vi "Model.vi"(0 "reference in":refnum<class "Battery.lvclass">, 5 "error in":errorcluster) -> (14 "reference out":refnum<class "Battery.lvclass">, 19 "error out":errorcluster)   [LabVIEW 2023, in "Battery.lvclass"]
uses:
  Battery.lvclass
  <vilib>/Utility/SystemLogging/NI_SystemLogging.lvlib
panel:
  out "Chart":dbl[][](graph)
  out "MODE":T1(ring)
  out "MODEL INDEX":i32
  out "error info":errorcluster
  out "Last Command":string
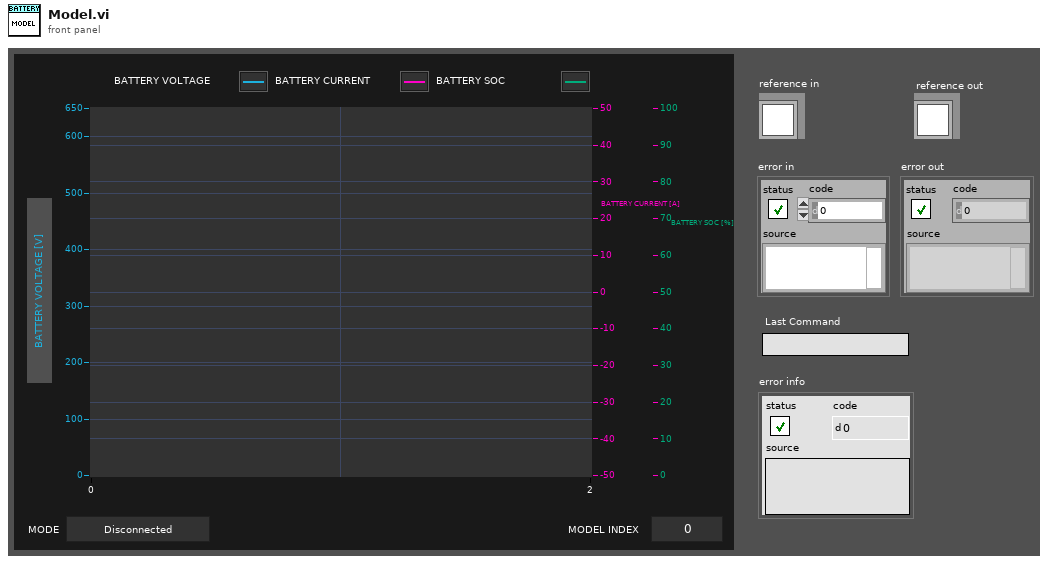
[diagram p1: front panel]
types:
  T1 = enum16{"Disconnected", "Charging", "Discharging"}
  T2 = cluster{"Core":cluster{"Timeout":i32, "Events":cluster{"EventsToProcess":refnum<event-registration>}, "EventFromProcess":refnum<user-event>, "ProcessSyncQueue":refnum<queue>, "QueueFromProcess":refnum<queue>, "Command":string, "Data":variant}}
  T3 = enum32{"Invalid", "Standard", "Closed", "Hidden", "Minimized", "Maximized"}
  T4 = cluster{"EventsToProcess":refnum<event-registration>}
  T5 = typedef "Battery.lvclass/ObjectAttributes.ctl" = cluster{"Mode":enum16{"Disconnected", "Charging", "Discharging"}, "Discharge Switch":bool, "Cell Voltage (V)":dbl, "Cell Current (A)":dbl, "SoC (%)":dbl, "Nominal Voltage (V)":dbl, "Model Index":i32}
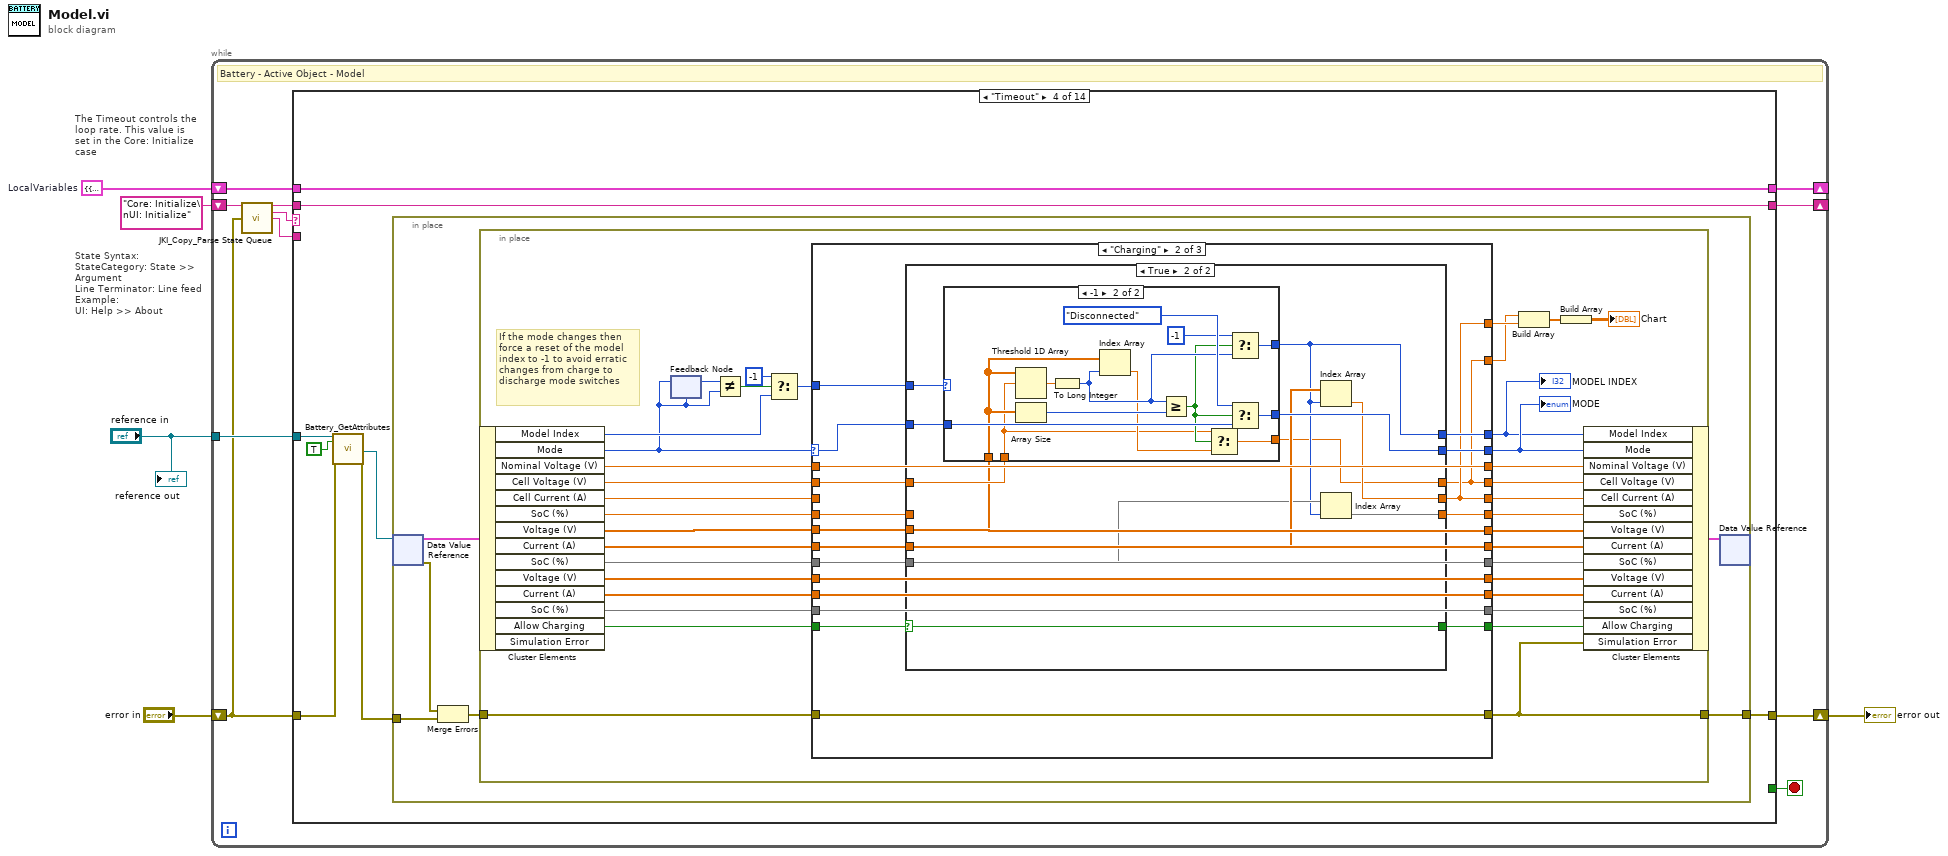
[diagram p0: block diagram]
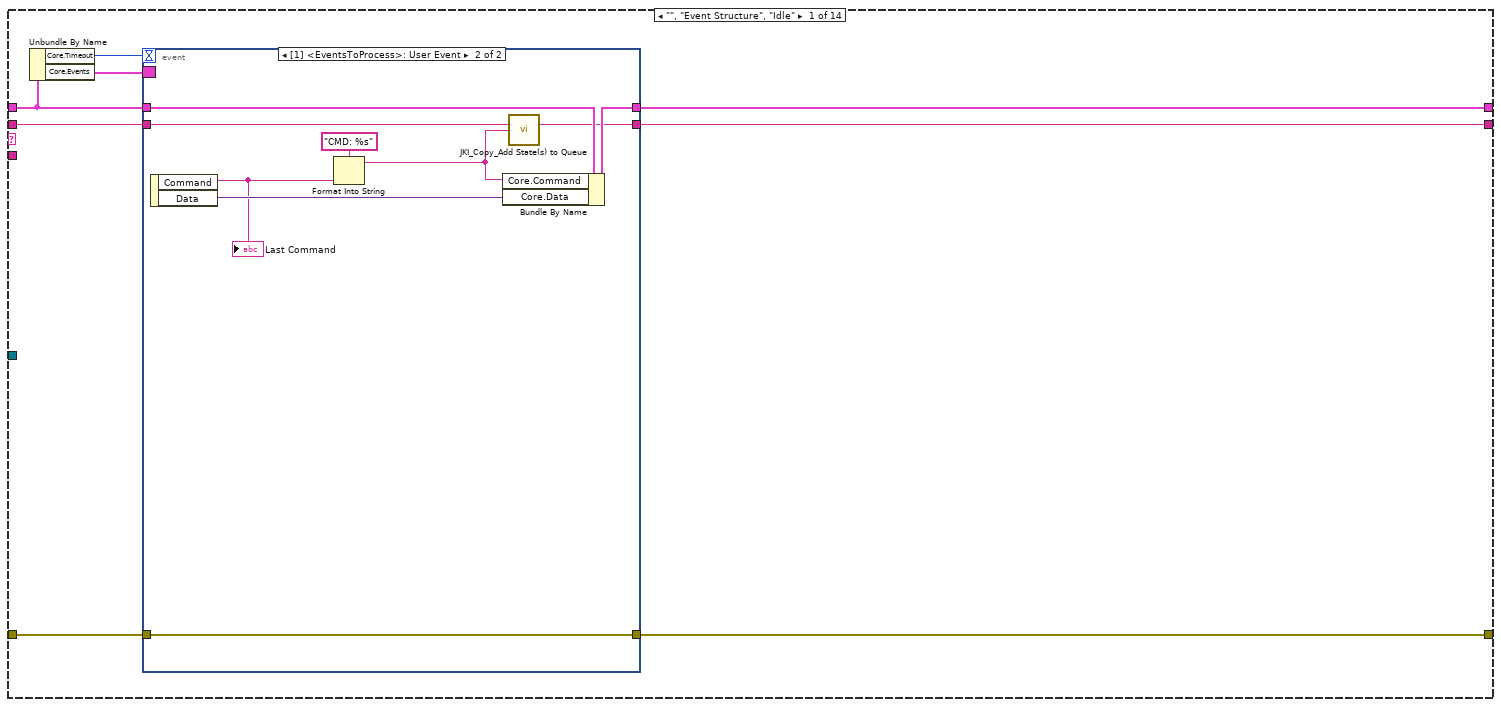
[diagram p2: hidden frame]
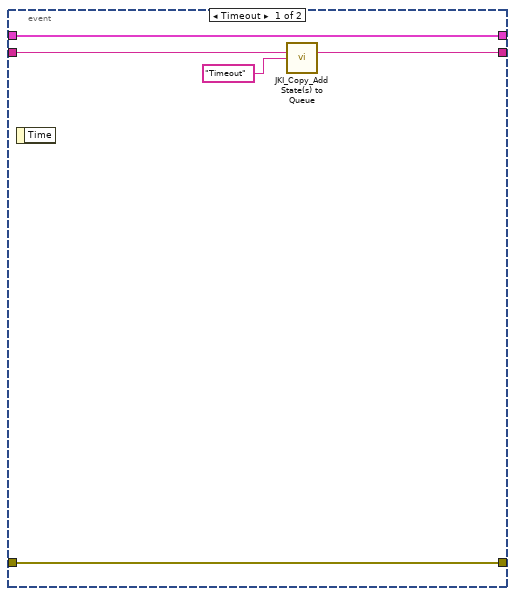
[diagram p3: hidden frame]
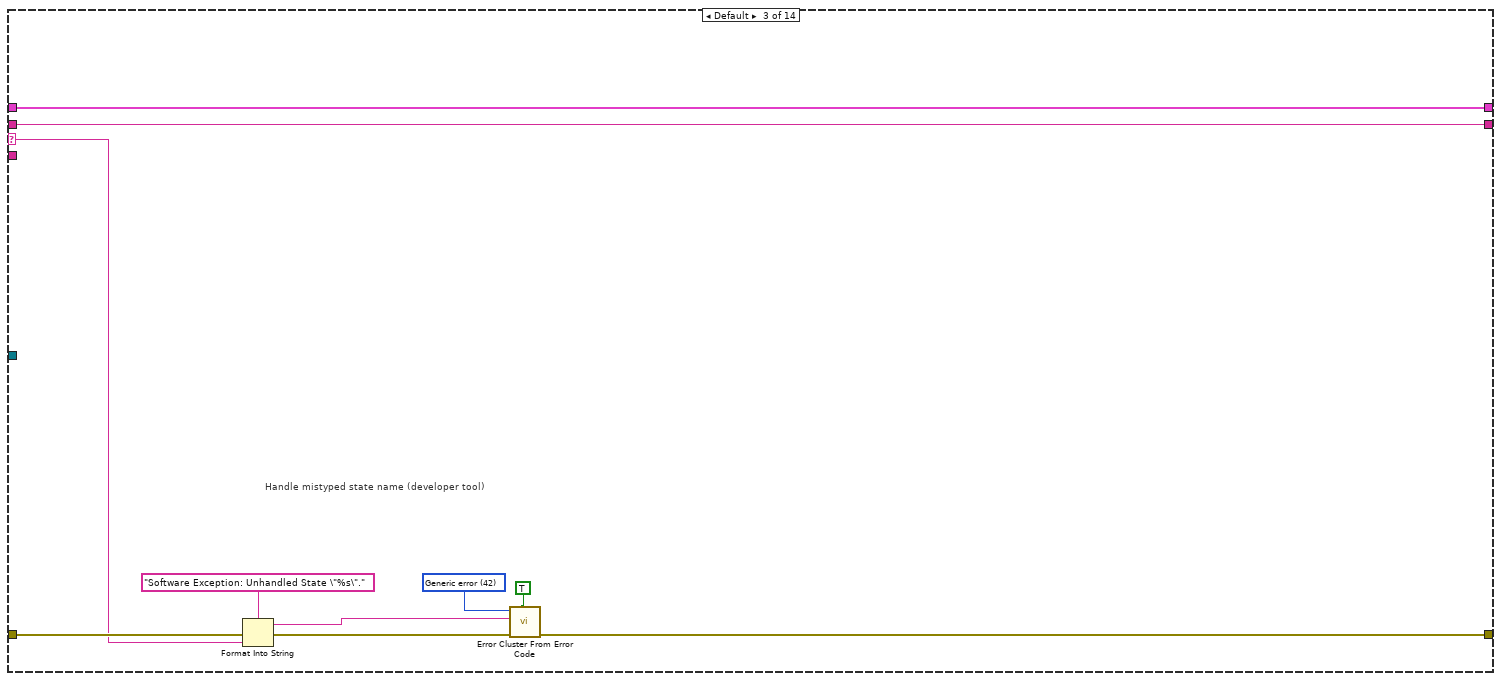
[diagram p5: hidden frame]
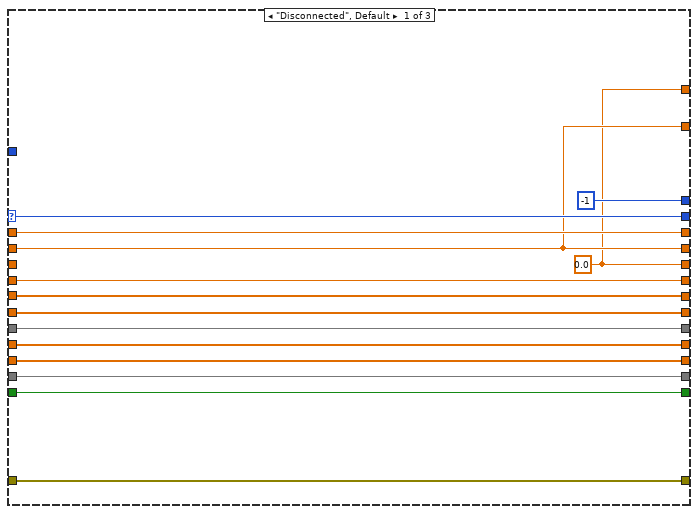
[diagram p6: hidden frame]
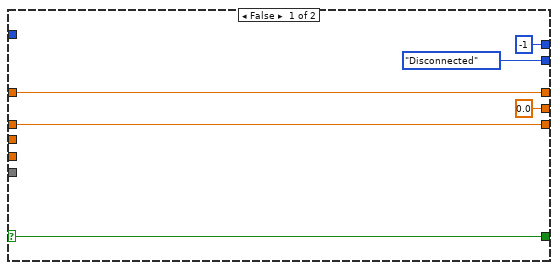
[diagram p7: hidden frame]
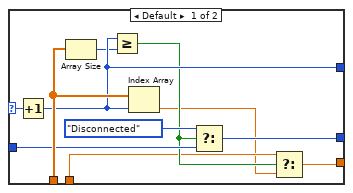
[diagram p8: hidden frame]
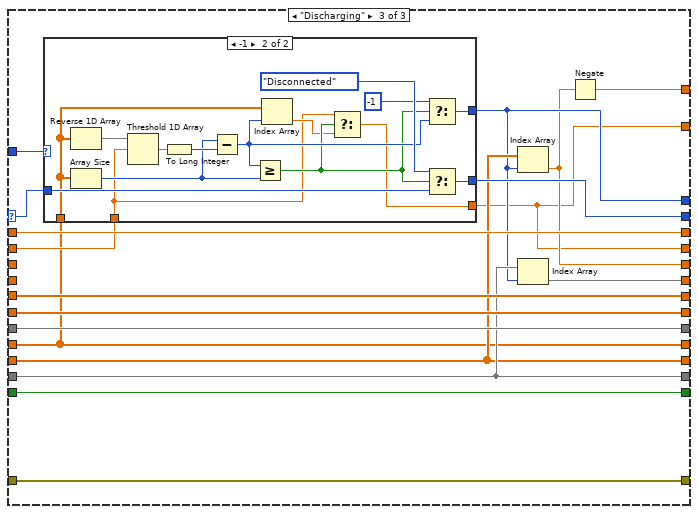
[diagram p9: hidden frame]
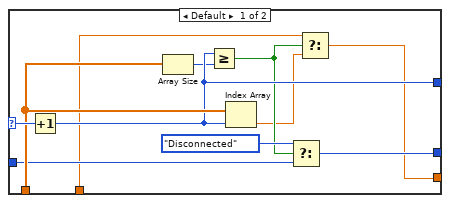
[diagram p10: hidden frame]
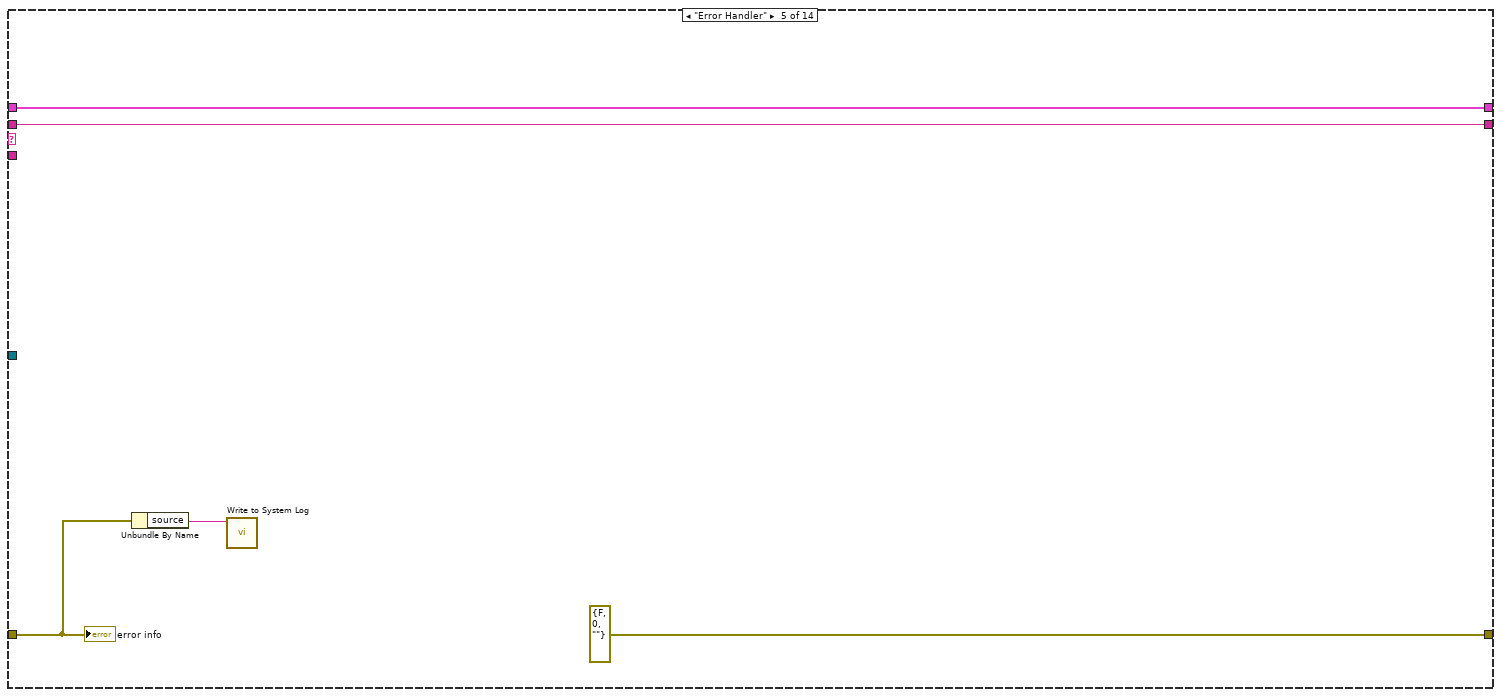
[diagram p11: hidden frame]
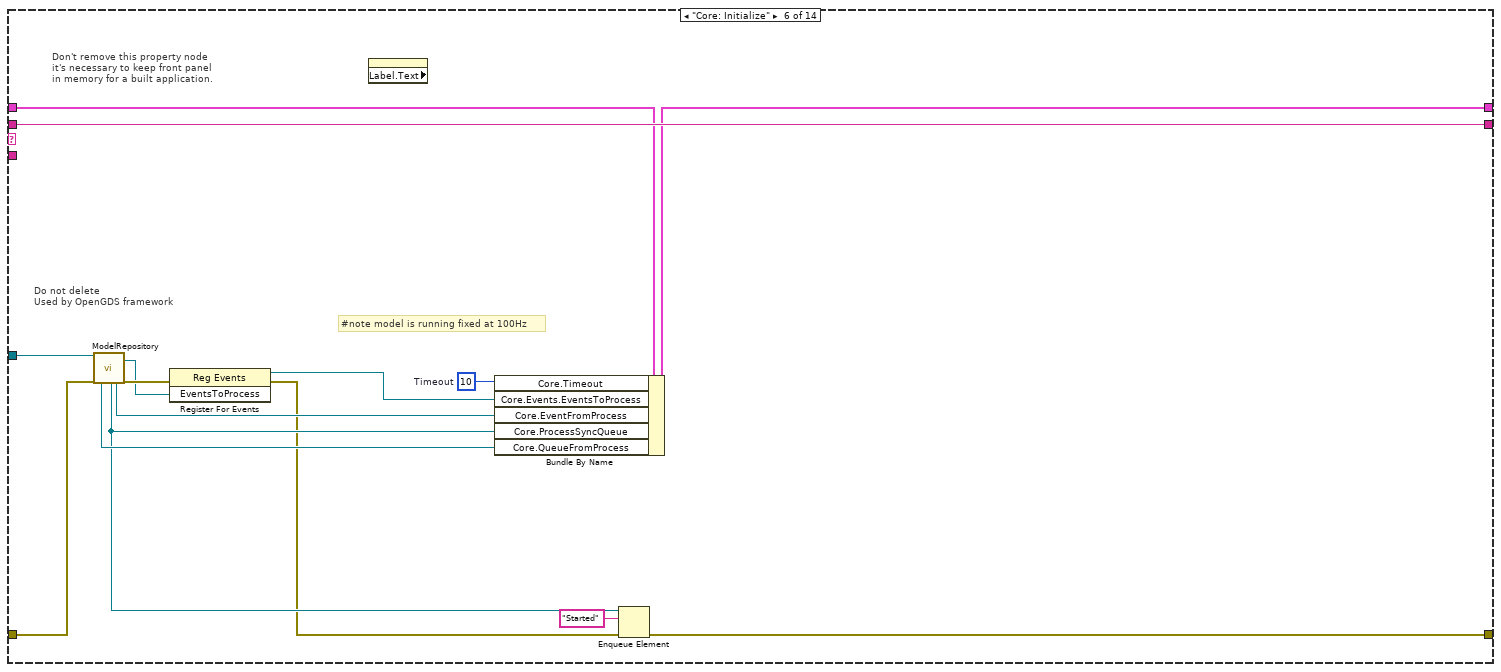
[diagram p12: hidden frame]
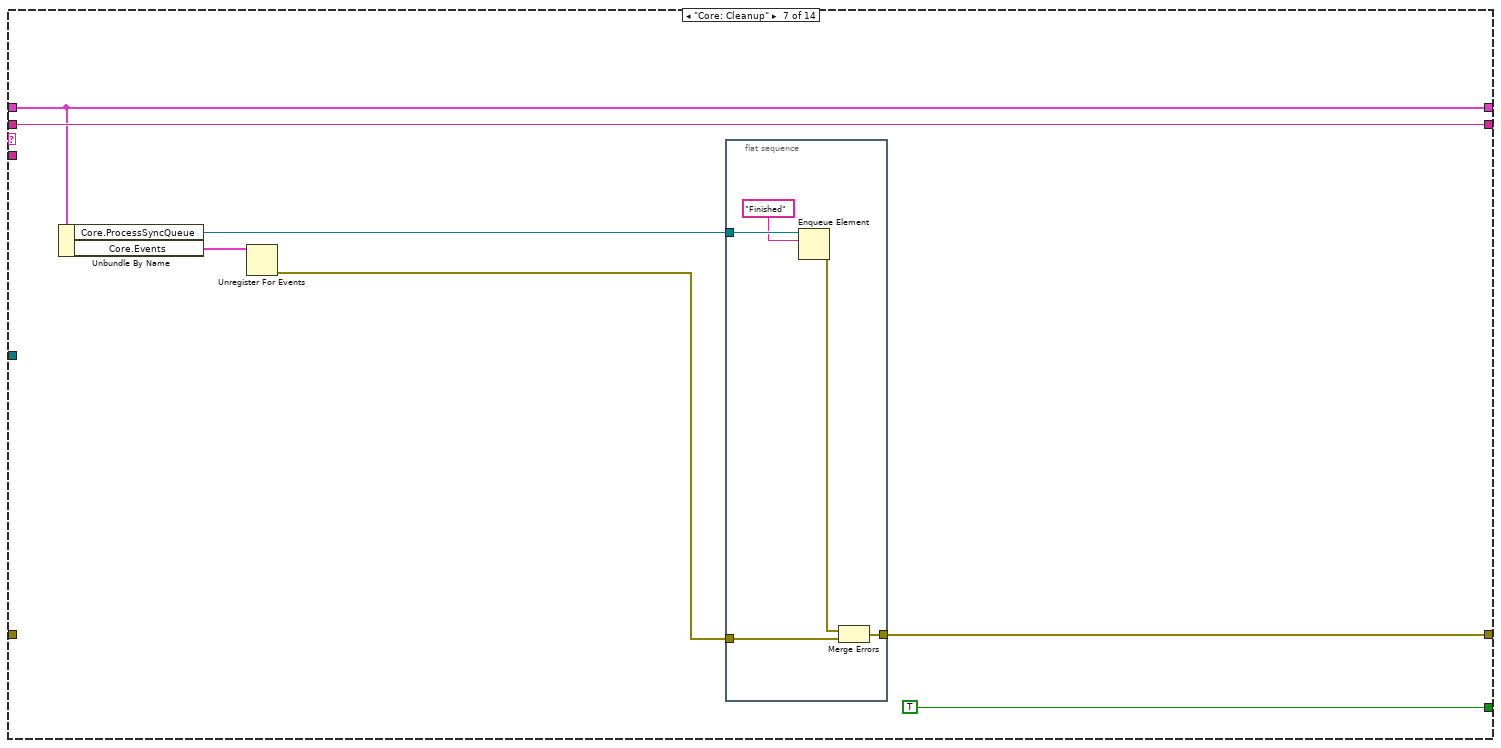
[diagram p13: hidden frame]
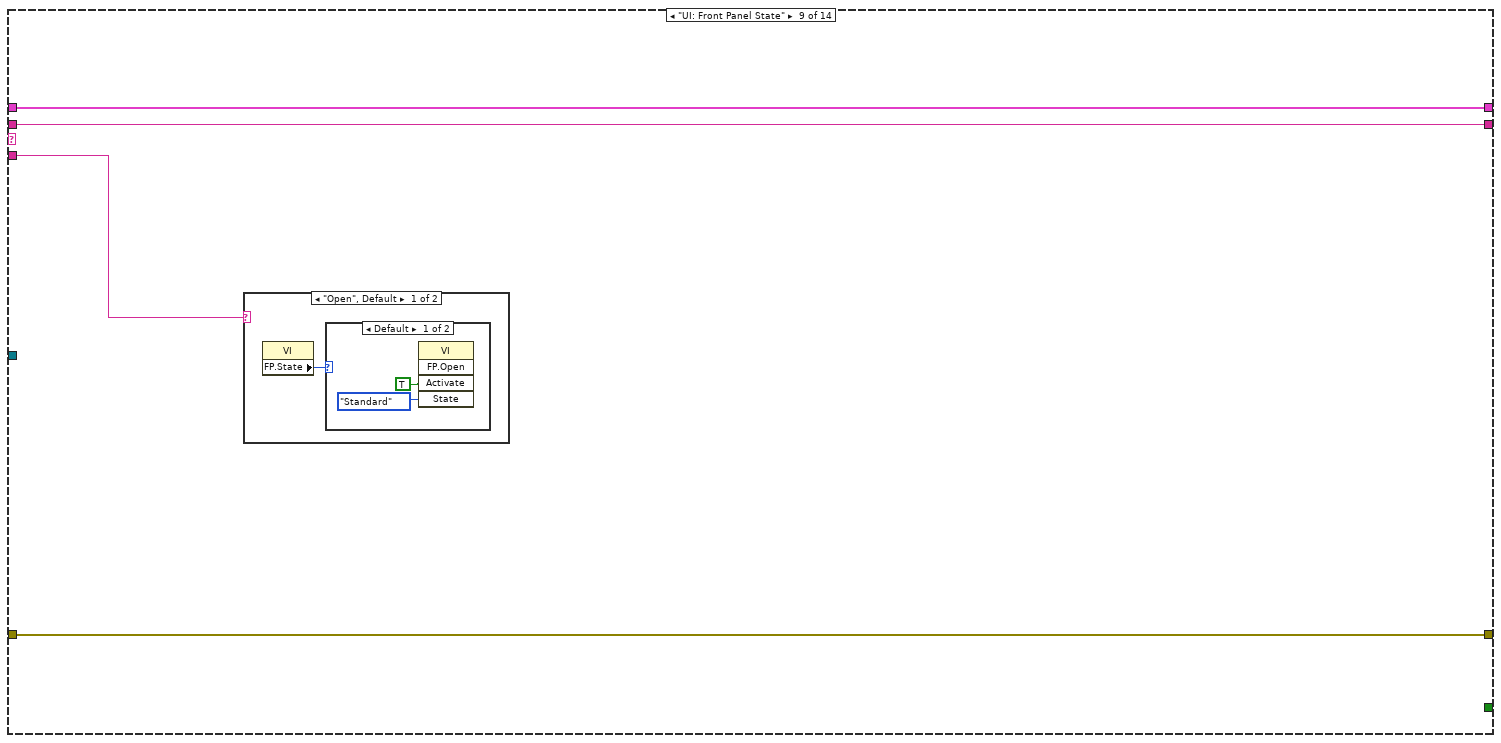
[diagram p15: hidden frame]
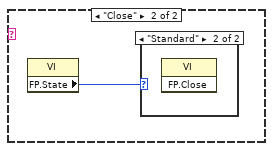
[diagram p17: hidden frame]
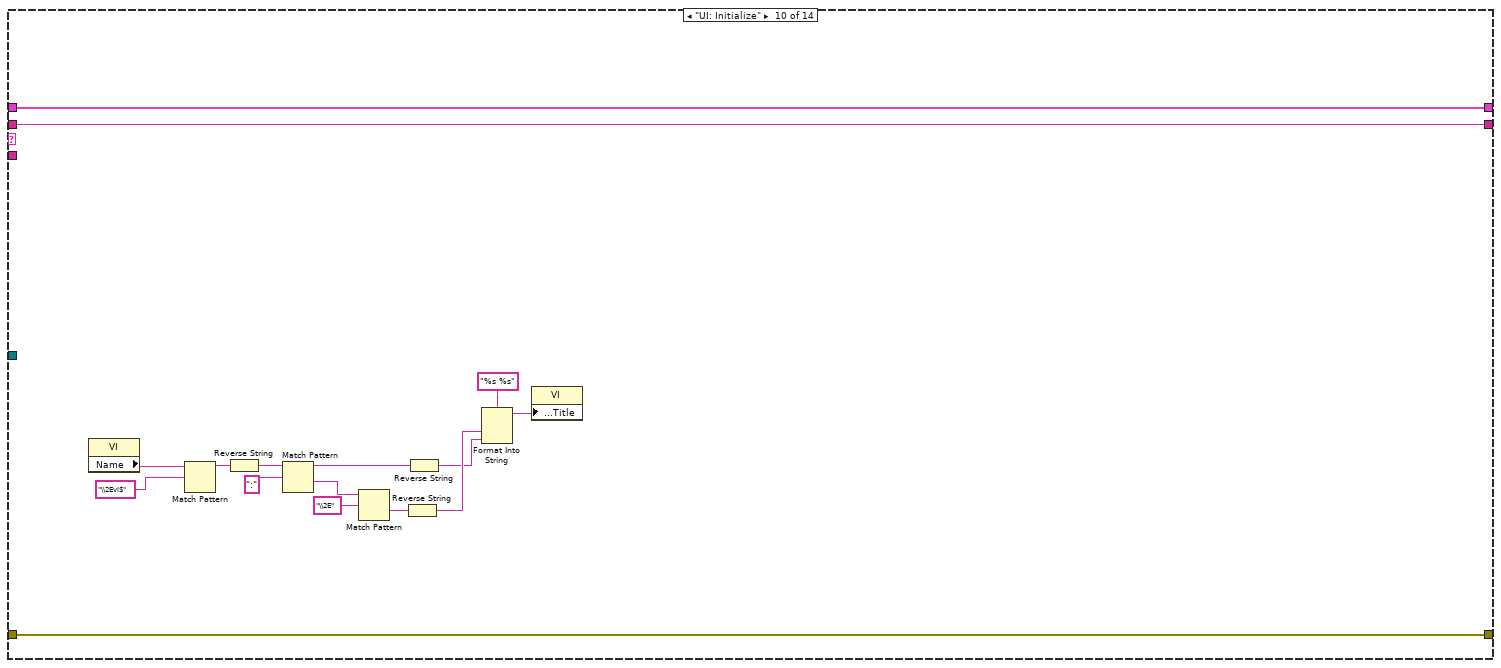
[diagram p19: hidden frame]
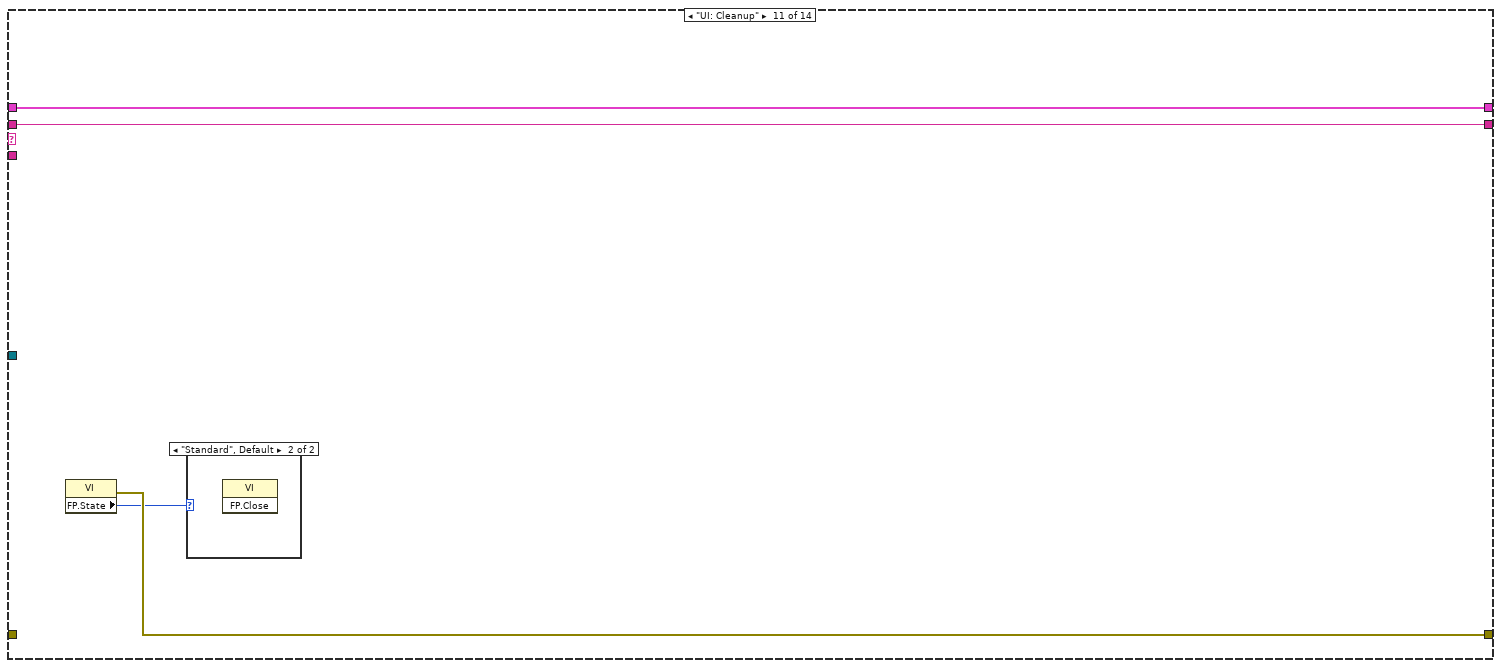
[diagram p20: hidden frame]
diagram:
  w5 = T2 {"Core"={"Timeout"=-1, "Events"={"EventsToProcess"=refnum}, "EventFromProcess"=refnum, "ProcessSyncQueue"=refnum, "QueueFromProcess"=refnum, "Command"="", "Data"=variant}}  # LocalVariables
  # "State Syntax:\nStateCategory: State >> Argument\nLine Terminator: Line feed\nExample:\nUI: Help >> About"
  # "The Timeout controls the loop rate. This value is set in the Core: Initialize case"
  n1 = while {
    shift-right: [w16] -> w4
    shift-left: "error in" -> [w6]
    shift-right: [w13] -> _
    shift-left: "Core: Initialize\nUI: Initialize" ("States Out") -> [w10]
    shift-right: [w15] -> _
    shift-left: w5 -> [w14]
    tunnel: "reference in" -> [w11]
    stop <- w12 stop-if-true
    # "Battery - Active Object - Model"
    n2 = call <vilib>:"JKI_Copy_Parse State Queue.vi"("State Queue"=w10, "Error In (no error)"=w6) -> ("Remaining States"=w9:string, "Current State"=w7:string, "Arguments"=w8:string)  [unwired: 11 in]
    n3 = case shown="\"Timeout\"" w7 {
      selector: w7 -> [_ _ w42 _ _ _ _ _ _ _ _ _ _ _]
      tunnel: w6 -> [w18 w41 w44 w57 w224 w226 _ w255 w256 w279 _ w286 w289 w296]
      tunnel: [w19 w41 w43 w53 errorcluster {"status"=FALSE, "code"=0, "source"=""} ("error constant") w240 w243 w255 w256 w279 w281 w286 w289 w296] -> w16
      tunnel: [w24 w40 w51 w55 w225 w238 w244 w254 w258 w277 w282 w285 w288 w295] -> w15
      tunnel: w14 -> [w20 w40 w51 w55 w225 w237 w244 w254 w258 w277 w282 w285 w288 w295]
      tunnel: w9 -> [w22 w39 w50 w56 w222 w239 w247 w253 w259 w278 w283 w284 _ w293]
      tunnel: w8 -> [_ _ _ _ _ _ _ _ w257 _ _ _ _ _]
      tunnel: [w21 w39 w50 w56 w222 w239 w247 w253 w259 w278 w283 w284 "UI: Cleanup\nCore: Cleanup" ("State(s) at Back (\"\")") w291] -> w13
      tunnel: [_ _ _ _ _ _ TRUE _ _ _ _ _ _ _] -> w12
      tunnel: w11 -> [_ _ _ w59 _ w227 _ _ _ _ _ _ _ _]
      frame "", "Event Structure", "Idle" {
        n4 = Unbundle By Name(w20) -> ("Core.Timeout"=w17:i32, "Core.Events"=w23:T4)
        n5 = event shown="[1] <EventsToProcess>: User Event" {
          selector: w23 -> [_ _]
          dyn-events: _ -> [_ _]
          timeout: w17 -> [_ _]
          tunnel: w20 -> [w29 w35]
          tunnel: [w29 w38] -> w24
          tunnel: [w26 w30] -> w21
          tunnel: w22 -> [w27 w31]
          tunnel: [w28 w36] -> w19
          tunnel: w18 -> [w28 w36]
          event Timeout {
            n6 = event-data() -> ()  [unwired: 1 in, 1 out]
            n7 = call <vilib>:"JKI_Copy_Add State(s) to Queue.vi"("State(s) in (\"\")"=w27, "State(s) at Back (\"\")"="Timeout" ("State(s) at Back (\"\")")) -> ("States Out"=w26:string)  [unwired: 13 in]
          }
          event User Event {
            n8 = event-data() -> ("Command"=w33:string, "Data"=w37:variant)  [unwired: 1 in]
            "Last Command" <- w33
            n9 = Format Into String(format string="CMD: %s", w33) -> (resulting string=w32:string)  [unwired: 2 in, 1 out]
            n10 = Bundle By Name(cluster=w35, "Core.Command"=w32, "Core.Data"=w37) -> (w38:T2)
            n11 = call <vilib>:"JKI_Copy_Add State(s) to Queue.vi"("State(s) in (\"\")"=w31, "State(s) at Back (\"\")"=w32) -> ("States Out"=w30:string)  [unwired: 13 in]
          }
        }
      }
      frame "---------- Core ----------" {
      }
      frame Default {
        w48 = 42 items=["No error", "Argument error", "Memory is full", "Out of zone", "End of file", "File already open", "Generic file I/O error", "File not found", "File permission error", "Disk is full", "Duplicate path", "Too many files open", "System feature not enabled", "Resource file not found", "Cannot add resource", "Resource not found", "Image not found", "Image memory error", "Pen does not exist", "Config type invalid", "Config token not found", "Config parse error", "Config memory error", "Bad external code format", "Bad external code offset", "External code not present", "Null window", "Destroy window error", "Null menu", "Print aborted", "Bad print record", "Print driver error", "Windows error during printing", "Memory error during printing", "Print dialog error", "Generic print error", "Invalid device refnum", "Device not found", "Device parameter error", "Device unit error", "Cannot open device", "Device call aborted", "Generic error", "Cancelled by user", "Object ID too low", "Object ID too high", "Object not in heap", "Unknown heap", "Unknown object (invalid DefProc)", "Unknown object (DefProc not in table)", "Message out of range", "Invalid (null) method", "Unknown message", "Manager call not supported", "Bad address", "Network operation in progress", "Network operation timed out", "Connection is busy", "Network attribute not supported", "Network error", "Address in use", "System out of memory", "Connection aborted", "Connection refused", "Not connected", "Already connected", "Connection closed", "Initialization error (interapplication manager)", "Bad occurrence", "Wait on unbound occurrence handler", "Occurrence queue overflow", "Datalog type conflict", "Unused", "Unrecognized type (interapplication manager)", "Memory corrupt", "Failed to make temporary DLL", "Old CIN version", "Drag socket not found", "Failed to load drop-object", "Failed to register OLE object", "Failed to release OLE object", "Format specifier type mismatch", "Unknown format specifier", "Too few format specifiers", "Too many format specifiers", "Scan failed", "Newer CIN version", "Error converting to variant", "Runtime menu error", "Password tampered", "Variant attribute not found", "Incompatible variant data type", "Event data is not available", "Event Store is not present", "Occurrence is not found", "Event Queue is not created", "Event info is not available", "Refnum passed is NULL", "Error retrieving Class GUID", "Error retrieving CoClass GUID", "Error retrieving TypeLib GUID.", "Bad built application magic bytes.", "Specific driver is different from the specific driver associated with the Logical Name.", "There is no session opened to the class driver.", "Max Error", "MAX - Error with config objects", "MAX - Error loading configuration", "MAX - Group not supported"]
        # "Handle mistyped state name (developer tool)"
        n12 = Format Into String(format string="Software Exception: Unhandled State \"%s\"." ("message"), error in=w44, w42) -> (resulting string=w47:string, error out=w46:errorcluster)  [unwired: 1 in]
        n13 = call <vilib>:"Error Cluster From Error Code.vi"("show call chain? (False)"=TRUE, "error in (no error)"=w46, "error message (\"\")"=w47, "error code (0)"=w48) -> ("error out"=w43:errorcluster)  [unwired: 5 in]
      }
      frame "Timeout" {
        n14 = call "Battery_GetAttributes.vi"("reference in"=w59, "OnlyGetDvrReference(False)"=TRUE, "Error In"=w57) -> ("DataRef"=w52:refnum<data-value>, "Error Out"=w54:errorcluster)  [unwired: 13 in, 2 out]
        n15 = in-place {
          in-place-border: w54 -> [w62]
          in-place-border: [w65] -> w53
          n16 = in-place-dvr #1(w52) -> (w64:T5, w60:errorcluster)
          n17 = Merge Errors(w60, w62) -> (w61:errorcluster)
          n18 = in-place {
            in-place-border: w61 -> [w101]
            in-place-border: [w66] -> w65
            # "If the mode changes then\nforce a reset of the model\nindex to -1 to avoid erratic\nchanges from charge to\ndischarge mode switches"
            n19 = in-place-cluster #2(w64) -> ("Model Index"=w83:i32, "Mode"=w80:T1, "Nominal Voltage (V)"=w96:dbl, "Cell Voltage (V)"=w100:dbl, "Cell Current (A)"=w99:dbl, "SoC (%)"=w97:dbl, "Voltage (V)"=w95:dbl[], "Current (A)"=w94:dbl[], "SoC (%)"=w93, "Voltage (V)"=w76:dbl[], "Current (A)"=w92:dbl[], "SoC (%)"=w91, "Allow Charging"=w68:bool)  [unwired: 1 out]
            n20 = feedback #3(w80) -> (w79:T1)
            n21 = feedback-in #3(w80) -> ()
            n22 = Not Equal?(x=w79, y=w80) -> (x != y?=w78:bool)
            n23 = Select(t=-1, s=w78, f=w83) -> (s? t:f=w82:i32)
            n24 = case shown="\"Charging\"" w80 {
              selector: w80 -> [w115 w127 w190]
              tunnel: [w115 w126 w189] -> w84
              tunnel: w101 -> [w114 w134 w194]
              tunnel: [w114 w134 w194] -> w66
              tunnel: w100 -> [w104 w129 w192]
              tunnel: [w104 w119 w178] -> w74
              tunnel: w99 -> [_ _ _]
              tunnel: [w103 w120 w180] -> w73
              tunnel: [w113 w123 w186] -> w98
              tunnel: w97 -> [w113 w116 _]
              tunnel: w96 -> [w112 w133 w193]
              tunnel: [w112 w133 w193] -> w75
              tunnel: w95 -> [w110 w121 w185]
              tunnel: w94 -> [w109 w125 w188]
              tunnel: w93 -> [w108 w124 w187]
              tunnel: w76 -> [w111 w132 w181]
              tunnel: w92 -> [w106 w131 w183]
              tunnel: w91 -> [w105 w130 w184]
              tunnel: [w111 w132 w181] -> w90
              tunnel: [w106 w131 w183] -> w89
              tunnel: [w105 w130 w184] -> w88
              tunnel: [w110 w121 w185] -> w87
              tunnel: w82 -> [_ w128 w191]
              tunnel: [-1 ("Model Index") w122 w182] -> w81
              tunnel: [w109 w125 w188] -> w86
              tunnel: [w108 w124 w187] -> w85
              tunnel: [w103 w120 w179] -> w70
              tunnel: [w104 w119 w178] -> w69
              tunnel: w68 -> [w102 w118 w177]
              tunnel: [w102 w117 w177] -> w67
              frame "Disconnected", Default {
                w103 = 0.0 ("Cell Current (A)")
                # "Maintain Voltage and SoC and set Current to 0A"
              }
              frame "Charging" {
                n25 = case shown="True" w118 {
                  selector: w118 -> [w135 w141]
                  tunnel: w129 -> [w138 w152]
                  tunnel: w128 -> [_ w151]
                  tunnel: w127 -> [_ w150]
                  tunnel: [T1."Disconnected" ("Mode") w149] -> w126
                  tunnel: w125 -> [_ w148]
                  tunnel: w124 -> [_ w147]
                  tunnel: [w140 w146] -> w123
                  tunnel: [-1 ("t") w145] -> w122
                  tunnel: w121 -> [_ w144]
                  tunnel: [0.0 w143] -> w120
                  tunnel: [w138 w142] -> w119
                  tunnel: [w135 w141] -> w117
                  tunnel: w116 -> [w140 _]
                  frame False {
                  }
                  frame True {
                    n26 = case shown="-1" w151 {
                      selector: w151 -> [w163 _]
                      tunnel: w144 -> [w162 w169]
                      tunnel: w152 -> [w155 w165]
                      tunnel: [w161 w172] -> w145
                      tunnel: [w153 w164] -> w142
                      tunnel: w150 -> [w159 w176]
                      tunnel: [w158 w174] -> w149
                      frame Default {
                        # "Increment until end of model.  Once model is finished, change mode to disconnect."
                        n27 = Increment(x=w163) -> (x+1=w161:i32)
                        n28 = Array Size(array=w162) -> (size(s)=w160:i32)
                        n29 = Greater Or Equal?(x=w161, y=w160) -> (x >= y?=w156:bool)
                        n30 = Index Array(array=w162, index=w161) -> (element=w154:dbl)
                        n31 = Select(t=T1."Disconnected", s=w156, f=w159) -> (s? t:f=w158:T1)
                        n32 = Select(t=w155, s=w156, f=w154) -> (s? t:f=w153:dbl)
                      }
                      frame -1 {
                        n33 = Threshold 1D Array(2:w165, 3:w169) -> (0:w170:dbl)  [unwired: 1 in]
                        n34 = Array Size(array=w169) -> (size(s)=w173:i32)
                        n35 = To Long Integer(number=w170) -> (32bit integer=w168:i32)
                        n36 = Index Array(array=w169, index=w168) -> (element=w167:dbl)
                        n37 = Greater Or Equal?(x=w168, y=w173) -> (x >= y?=w166:bool)
                        n38 = Select(t=w165, s=w166, f=w167) -> (s? t:f=w164:dbl)
                        n39 = Select(t=-1, s=w166, f=w168) -> (s? t:f=w172:i32)
                        n40 = Select(t=T1."Disconnected", s=w166, f=w176) -> (s? t:f=w174:T1)
                      }
                    }
                    n41 = Index Array(array=w148, index=w145) -> (element=w143:dbl)
                    n42 = Index Array(array=w147, index=w145) -> (element=w146)
                  }
                }
              }
              frame "Discharging" {
                n43 = case shown="-1" w191 {
                  selector: w191 -> [w205 _]
                  tunnel: w181 -> [w204 w214]
                  tunnel: w192 -> [w197 w207]
                  tunnel: [w203 w217] -> w182
                  tunnel: [w195 w206] -> w178
                  tunnel: w190 -> [w201 w220]
                  tunnel: [w200 w218] -> w189
                  frame Default {
                    # "Increment until end of model.  Once model is finished, change mode to disconnect."
                    n44 = Increment(x=w205) -> (x+1=w203:i32)
                    n45 = Array Size(array=w204) -> (size(s)=w202:i32)
                    n46 = Greater Or Equal?(x=w203, y=w202) -> (x >= y?=w198:bool)
                    n47 = Index Array(array=w204, index=w203) -> (element=w196:dbl)
                    n48 = Select(t=T1."Disconnected", s=w198, f=w201) -> (s? t:f=w200:T1)
                    n49 = Select(t=w197, s=w198, f=w196) -> (s? t:f=w195:dbl)
                  }
                  frame -1 {
                    # "Check for next voltage in the array, or if the voltage is already full charge, then go to disconnected state."
                    n50 = Reverse 1D Array(array=w214) -> (reversed array=w213:dbl[])
                    n51 = Array Size(array=w214) -> (size(s)=w211:i32)
                    n52 = Threshold 1D Array(2:w207, 3:w213) -> (0:w215:dbl)  [unwired: 1 in]
                    n53 = To Long Integer(number=w215) -> (32bit integer=w212:i32)
                    n54 = Subtract(x=w211, y=w212) -> (x-y=w210:i32)
                    n55 = Greater Or Equal?(x=w210, y=w211) -> (x >= y?=w209:bool)
                    n56 = Index Array(array=w214, index=w210) -> (element=w208:dbl)
                    n57 = Select(t=w207, s=w209, f=w208) -> (s? t:f=w206:dbl)
                    n58 = Select(t=-1, s=w209, f=w210) -> (s? t:f=w217:i32)
                    n59 = Select(t=T1."Disconnected", s=w209, f=w220) -> (s? t:f=w218:T1)
                  }
                }
                n60 = Index Array(array=w183, index=w182) -> (element=w180:dbl)
                n61 = Index Array(array=w184, index=w182) -> (element=w186)
                n62 = Negate(x=w180) -> (-x=w179:dbl)
              }
            }
            "MODEL INDEX" <- w81
            "MODE" <- w84
            n63 = Build Array(w69, w70) -> (w72:dbl[])
            n64 = Build Array(w72) -> (→"Chart":dbl[][])
            n65 = in-place-cluster #2("Model Index"=w81, "Mode"=w84, "Nominal Voltage (V)"=w75, "Cell Voltage (V)"=w74, "Cell Current (A)"=w73, "SoC (%)"=w98, "Voltage (V)"=w87, "Current (A)"=w86, "SoC (%)"=w85, "Voltage (V)"=w90, "Current (A)"=w89, "SoC (%)"=w88, "Allow Charging"=w67, "Simulation Error"=w66) -> (w63:T5)
          }
          n66 = in-place-dvr #1(w63) -> ()  [unwired: 2 out]
        }
      }
      frame "Error Handler" {
        n67 = Unbundle By Name(w224) -> ("source"=w221:string)
        n68 = call <vilib>:"Write to System Log.vi"("message"=w221) -> ()  [unwired: 10 in, 1 out]
        "error info" <- w224
      }
      frame "Core: Initialize" {
        w228 = 10  # Timeout
        # "#note model is running fixed at 100Hz"
        # "Do not delete\nUsed by OpenGDS framework"
        # "Don't remove this property node\nit's necessary to keep front panel\nin memory for a built application."
        # "Template created by VI Technologies"
        n69 = call "ModelRepository.vi"("reference in"=w227, "Error In"=w226) -> ("QueueFromProcess"=w232:refnum<queue>, "ProcessSyncQueue"=w230:refnum<queue>, "EventFromProcess"=w233:refnum<user-event>, "EventsToProcess"=w235:refnum<user-event>, "Error Out"=w236:errorcluster)  [unwired: 10 in, 3 out]
        n70 = register-events(error in=w236, w235) -> (reference out=w234:refnum<event-registration>, error out=w229:errorcluster)  [unwired: 1 in]
        n71 = property on="reference in" class="LVClassControl (strict)" props=["Label", "Text"]() -> ()  [unwired: 2 in, 3 out]
        n72 = Bundle By Name(cluster=w237, "Core.Timeout"=w228, "Core.Events.EventsToProcess"=w234, "Core.EventFromProcess"=w233, "Core.ProcessSyncQueue"=w230, "Core.QueueFromProcess"=w232) -> (w238:T2)
        n73 = Enqueue Element(queue=w230, element="Started", error in (no error)=w229) -> (error out=w240:errorcluster)  [unwired: 1 in, 2 out]
      }
      frame "Core: Cleanup" {
        n74 = Unbundle By Name(w244) -> ("Core.ProcessSyncQueue"=w245:refnum<queue>, "Core.Events"=w242:T4)
        n75 = Unregister For Events(event registration refnum=w242) -> (error out=w241:errorcluster)  [unwired: 1 in]
        n76 = flat-sequence {
          tunnel: [w251] -> w243
          tunnel: w245 -> [w250]
          tunnel: w241 -> [w249]
          frame #0 {
            n77 = Enqueue Element(queue=w250, element="Finished") -> (error out=w252:errorcluster)  [unwired: 2 in, 2 out]
            n78 = Merge Errors(w252, w249) -> (w251:errorcluster)
          }
        }
      }
      frame "---------- UI ----------" {
      }
      frame "UI: Front Panel State" {
        n79 = case shown="\"Open\", Default" w257 {
          frame "Open", Default {
            n80 = property class="VI"() -> ("FP.State"=w260:T3)  [unwired: 2 in, 2 out]
            n81 = case shown="Default" w260 {
              frame Default {
                n82 = invoke class="VI" method="FP.Open"("Activate"=TRUE, "State"=T3."Standard") -> ()  [unwired: 3 in, 5 out]
              }
              frame "Standard" {
              }
            }
          }
          frame "Close" {
            n83 = property class="VI"() -> ("FP.State"=w263:T3)  [unwired: 2 in, 2 out]
            n84 = case shown="\"Standard\"" w263 {
              frame Default {
              }
              frame "Standard" {
                n85 = invoke class="VI" method="FP.Close"() -> ()  [unwired: 3 in, 3 out]
              }
            }
          }
        }
      }
      frame "UI: Initialize" {
        n86 = property class="VI"() -> ("Name"=w276:string)  [unwired: 2 in, 2 out]
        n87 = Match Pattern(string=w276, regular expression="\\2Evi$") -> (before substring=w274:string)  [unwired: 1 in, 3 out]
        n88 = Reverse String(1:w274) -> (0:w273:string)
        n89 = Match Pattern(string=w273, regular expression=":") -> (before substring=w271:string, after substring=w270:string)  [unwired: 1 in, 2 out]
        n90 = Match Pattern(string=w270, regular expression="\\2E") -> (after substring=w268:string)  [unwired: 1 in, 3 out]
        n91 = Reverse String(1:w268) -> (0:w267:string)
        n92 = Reverse String(1:w271) -> (0:w266:string)
        n93 = Format Into String(format string="%s %s", w267, w266) -> (resulting string=w265:string)  [unwired: 2 in, 1 out]
        n94 = property class="VI"("Front Panel.Title"=w265) -> ()  [unwired: 2 in, 2 out]
      }
      frame "UI: Cleanup" {
        n95 = property class="VI"() -> (error out=w281:errorcluster, "FP.State"=w280:T3)  [unwired: 2 in, 1 out]
        n96 = case shown="\"Standard\", Default" w280 {
          frame "Closed" {
          }
          frame "Standard", Default {
            n97 = invoke class="VI" method="FP.Close"() -> ()  [unwired: 3 in, 3 out]
          }
        }
      }
      frame "-------- CMD --------" {
      }
      frame "CMD: Exit" {
      }
      frame "CMD: Front Panel State" {
        n98 = Format Into String(format string="UI: Front Panel State>>%s" ("string"), "Open" ("input 1")) -> (resulting string=w292:string)  [unwired: 2 in, 1 out]
        n99 = call <vilib>:"JKI_Copy_Add State(s) to Queue.vi"("State(s) in (\"\")"=w293, "State(s) at Back (\"\")"=w292) -> ("States Out"=w291:string)  [unwired: 13 in]
      }
    }
  }
  "error out" <- w4
  "reference out" <- "reference in"
